vi "Periodic Tasks.vi"(8 "error in":errorcluster) -> ()   [LabVIEW 2017]
doc: "This VI runs in parallel to other tasks. It can contain as many user-defined periodic loops as you need. These can carry out PID or other sorts of timed response."
uses:
  <vilib>/Rock Robotics/WPI/Utilities/WPI_GetSetVariantRefNum.vi
  Robot Global Data.vi
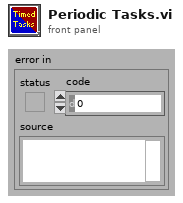
[diagram p1: front panel]
types:
  T1 = typedef "WPI_JoystickDevRef.ctl" = cluster{"Device":T2}
  T2 = typedef "WPI_JoystickDeviceEnum.ctl" = enum16{"USB 0", "USB 1", "USB 2", "USB 3", "USB 4", "USB 5"}
  T3 = typedef "WPI_RobotDriveDevRef.ctl" = cluster{"DevStatus":errorcluster, "Motors[]":T4[], "Square Inputs":bool, "Max Output":dbl}
  T4 = typedef "WPI_MotorControlDeviceRef.ctl" = cluster{"DeviceStatus":errorcluster, "Type":T5, "PWM":cluster{"PWM Channel":T6, "DeadBand":T7}, "CAN":cluster{"Device Number":u8, "SetOutput VI Ref":variant, "GetOutput VI Ref":variant, "Enable VI Ref":variant, "Disable VI Ref":variant, "Data":variant}, "Invert":bool, "DIO PWM":cluster{"PWM \"Enable\" Channel":T6, "DIOChannel":T8, "PWM Rate":dbl}}
  T5 = typedef "WPI_MotorControlType.ctl" = enum16{"PWM", "CAN", "DIO PWM"}
  T6 = typedef "FPGA_DIOPWMChannel.ctl" = enum8{"PWM 0", "PWM 1", "PWM 2", "PWM 3", "PWM 4", "PWM 5", "PWM 6", "PWM 7", "PWM 8", "PWM 9", "PWM MXP 0", "PWM MXP 1", "PWM MXP 2", "PWM MXP 3", "PWM MXP 4", "PWM MXP 5", "PWM MXP 6", "PWM MXP 7", "PWM MXP 8", "PWM MXP 9", "Invalid"}
  T7 = typedef "WPI_PWMDeadband.ctl" = cluster{"Name":string, "maxPositivePwm":i32, "minPositivePwm":i32, "centerPwm":i32, "maxNegativePwm":i32, "minNegativePwm":i32, "angularRange":u16}
  T8 = typedef "FPGA_DIOChannel.ctl" = enum8{"DIO 0", "DIO 1", "DIO 2", "DIO 3", "DIO 4", "DIO 5", "DIO 6", "DIO 7", "DIO 8", "DIO 9", "DIO MXP 0", "DIO MXP 1", "DIO MXP 2", "DIO MXP 3", "DIO MXP 4", "DIO MXP 5", "DIO MXP 6", "DIO MXP 7", "DIO MXP 8", "DIO MXP 9", "DIO MXP 10", "DIO MXP 11", "DIO MXP 12", "DIO MXP 13", "DIO MXP 14", "DIO MXP 15", "SPI Port CS1", "SPI Port CS2", "SPI Port CS3", "SPI Port MISO", "SPI Port MOSI", "Invalid"}
  T9 = typedef "WPI_EncoderDevRef.ctl" = cluster{"DevStatus":errorcluster, "EncoderIndex":T10, "CounterIndex":T11, "DistancePerCount":dbl, "Decoding Type":T12}
  T10 = typedef "FPGA_EncoderIdx.ctl" = enum8{"Enc 0", "Enc 1", "Enc 2", "Enc 3", "Enc 4", "Enc 5", "Enc 6", "Enc 7", "Invalid"}
  T11 = typedef "FPGA_CounterCtrSystemIndex.ctl" = enum8{"Ctr 0", "Ctr 1", "Ctr 2", "Ctr 3", "Ctr 4", "Ctr 5", "Ctr 6", "Ctr 7", "Invalid"}
  T12 = typedef "WPI_EncoderType.ctl" = enum16{"1x", "2x", "4x"}
  T13 = cluster{"JoystickDevRef":T1, "RobotDriveDevRef":T3}
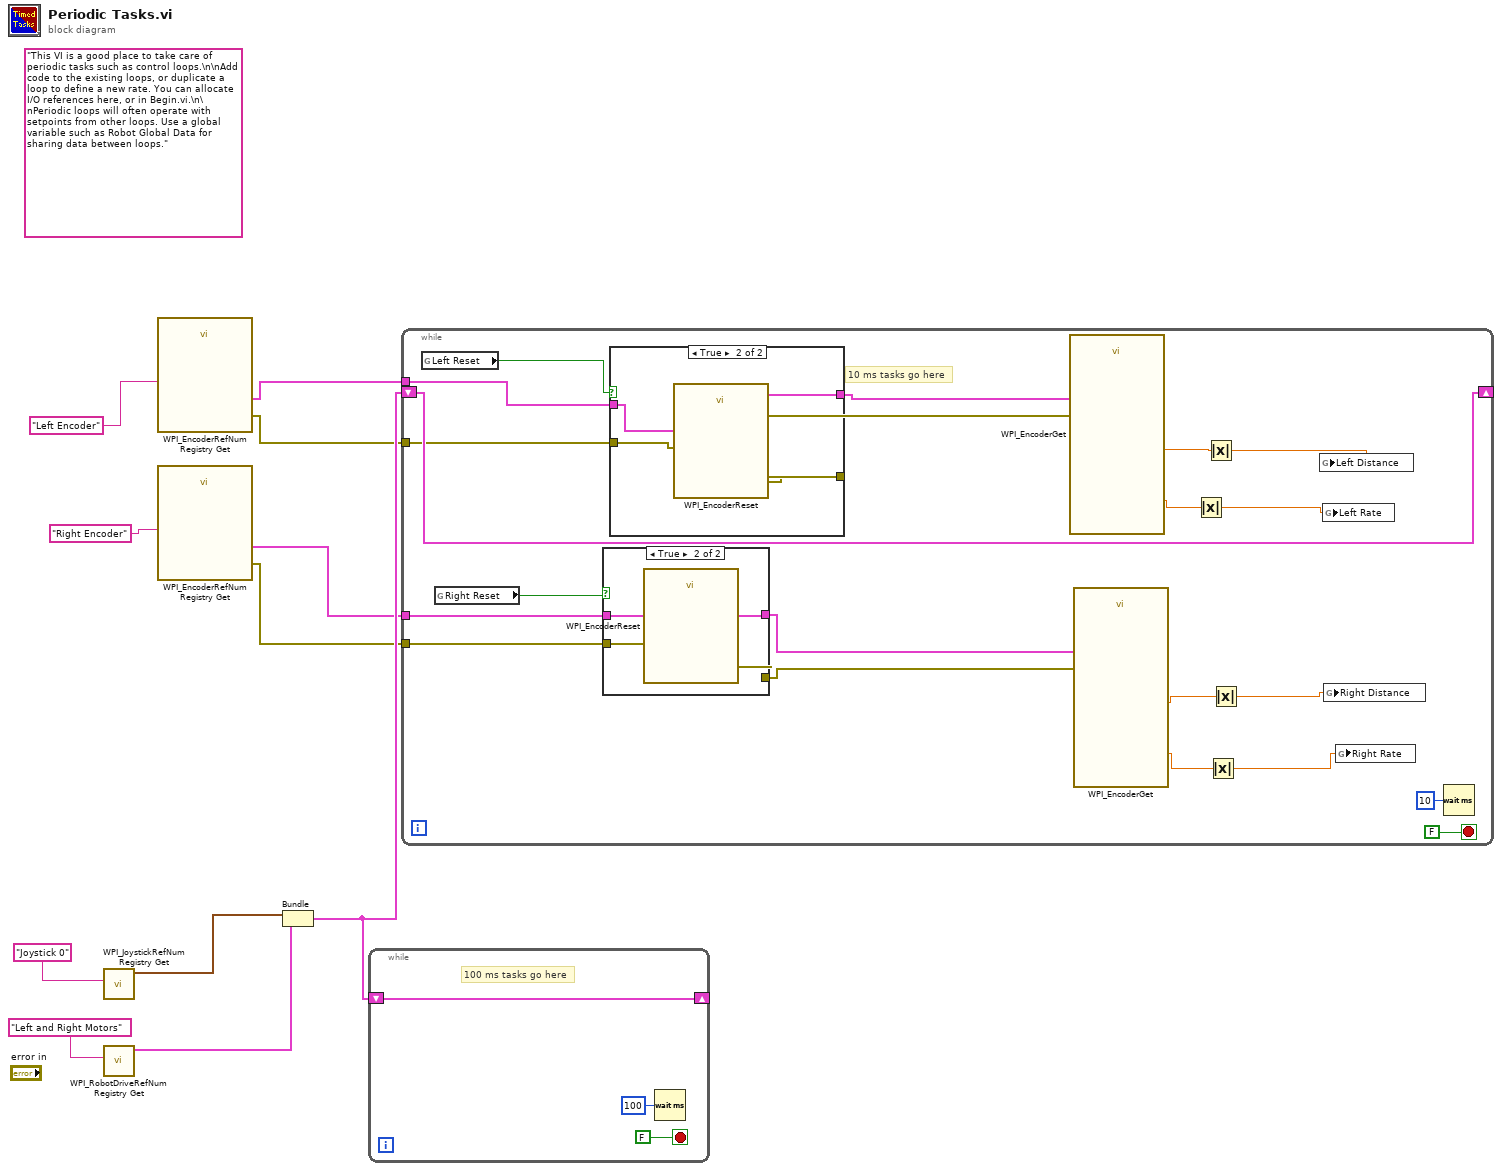
[diagram p0: block diagram]
diagram:
  (unwired) "This VI is a good place to take care of periodic tasks such as control loops.\n\nAdd code to the existing loops, or duplicate a loop to define a new rate. You can allocate I/O references here, or in Begin.vi.\n\nPeriodic loops will often operate with setpoints from other loops. Use a global variable such as Robot Global Data for sharing data between loops."
  n1 = call <vilib>:"WPI_JoystickRefNum Registry Get.vi"("refnum name"="Joystick 0") -> ("JoystickDevRef"=w9:T1)  [unwired: 1 in, 9 out]
  n2 = call <vilib>:"WPI_RobotDriveRefNum Registry Get.vi"("refnum name"="Left and Right Motors") -> ("RobotDriveDevRef"=w8:T3)  [unwired: 1 in, 9 out]
  n3 = call <vilib>:"WPI_EncoderRefNum Registry Get.vi"("refnum name"="Left Encoder") -> ("error out"=w1:errorcluster, "EncoderDevRef"=w2:T9)  [unwired: 9 in]
  n4 = call <vilib>:"WPI_EncoderRefNum Registry Get.vi"("refnum name"="Right Encoder") -> ("error out"=w4:errorcluster, "EncoderDevRef"=w3:T9)  [unwired: 9 in]
  n5 = Bundle("JoystickDevRef"=w9, "RobotDriveDevRef"=w8) -> (w7:T13)  [unwired: 1 out]
  n6 = while {
    shift-right: [w12] -> _
    shift-left: w7 -> [w12]
    stop <- FALSE stop-if-true
    # "100 ms tasks go here"
    n7 = Wait (ms)(milliseconds to wait=u32 100) -> ()  [unwired: 1 out]
  }
  n8 = while {
    shift-right: [w33] -> _
    shift-left: w7 -> [w33]
    tunnel: w4 -> [w32]
    tunnel: w3 -> [w31]
    tunnel: w2 -> [w28]
    tunnel: w1 -> [w27]
    stop <- FALSE stop-if-true
    # "10 ms tasks go here"
    n9 = global read "Robot Global Data.vi" "Left Reset"() -> (w24:bool)
    n10 = global read "Robot Global Data.vi" "Right Reset"() -> (w23:bool)
    n11 = case shown="True" w23 {
      tunnel: [w43 w47] -> w30
      tunnel: w32 -> [w42 w46]
      tunnel: [w42 w45] -> w29
      tunnel: w31 -> [w43 w44]
      frame False {
      }
      frame True {
        n12 = call <vilib>:"WPI_EncoderReset.vi"("error in (no error)"=w46, "EncoderDevRef"=w44) -> ("error out"=w45:errorcluster, "EncoderDevRef"=w47:T9)  [unwired: 8 in]
      }
    }
    n13 = case shown="True" w24 {
      tunnel: [w37 w41] -> w26
      tunnel: w28 -> [w37 w40]
      tunnel: w27 -> [w36 w39]
      tunnel: [w36 w38] -> w25
      frame False {
      }
      frame True {
        n14 = call <vilib>:"WPI_EncoderReset.vi"("error in (no error)"=w39, "EncoderDevRef"=w40) -> ("error out"=w38:errorcluster, "EncoderDevRef"=w41:T9)  [unwired: 8 in]
      }
    }
    n15 = call <vilib>:"WPI_EncoderGet.vi"("error in (no error)"=w25, "EncoderDevRef"=w26) -> ("Distance"=w22:dbl, "Rate"=w20:dbl)  [unwired: 4 in, 4 out]
    n16 = call <vilib>:"WPI_EncoderGet.vi"("error in (no error)"=w29, "EncoderDevRef"=w30) -> ("Distance"=w18:dbl, "Rate"=w16:dbl)  [unwired: 4 in, 4 out]
    n17 = Absolute Value(x=w20) -> (abs(x)=w19:dbl)
    n18 = Absolute Value(x=w22) -> (abs(x)=w21:dbl)
    n19 = Absolute Value(x=w16) -> (abs(x)=w15:dbl)
    n20 = Absolute Value(x=w18) -> (abs(x)=w17:dbl)
    n21 = global write "Robot Global Data.vi" "Left Distance"(w21) -> ()
    n22 = global write "Robot Global Data.vi" "Left Rate"(w19) -> ()
    n23 = global write "Robot Global Data.vi" "Right Distance"(w17) -> ()
    n24 = global write "Robot Global Data.vi" "Right Rate"(w15) -> ()
    n25 = Wait (ms)(milliseconds to wait=u32 10) -> ()  [unwired: 1 out]
  }
